vi "readAmbient.vi"() -> ()   [LabVIEW 2011]
uses:
  <vilib>/Utility/file.llb/Read From Spreadsheet File (string).vi
panel:
  out "Table Control":string[][](table)
  in  "EXIT":bool
  in  "OK Button":bool
  in  "Boolean":bool caption="Choose date    Today"
  out "Diff Press":cluster{dbl[], dbl[]}(graph)
  out "Press":cluster{dbl[], dbl[]}(graph)
  out "Umidity":cluster{dbl[], dbl[]}[](graph)=[{[1.0, 2.0, 4.0], [2.0, 1.0, 0.0]}, {[0.5, 1.5, 3.5], [3.0, 4.0, 2.0]}]
  out "Temperature":cluster{dbl[], dbl[]}[](graph)=[{[1.0, 2.0, 4.0], [2.0, 1.0, 0.0]}, {[0.5, 1.5, 3.5], [3.0, 4.0, 2.0]}]
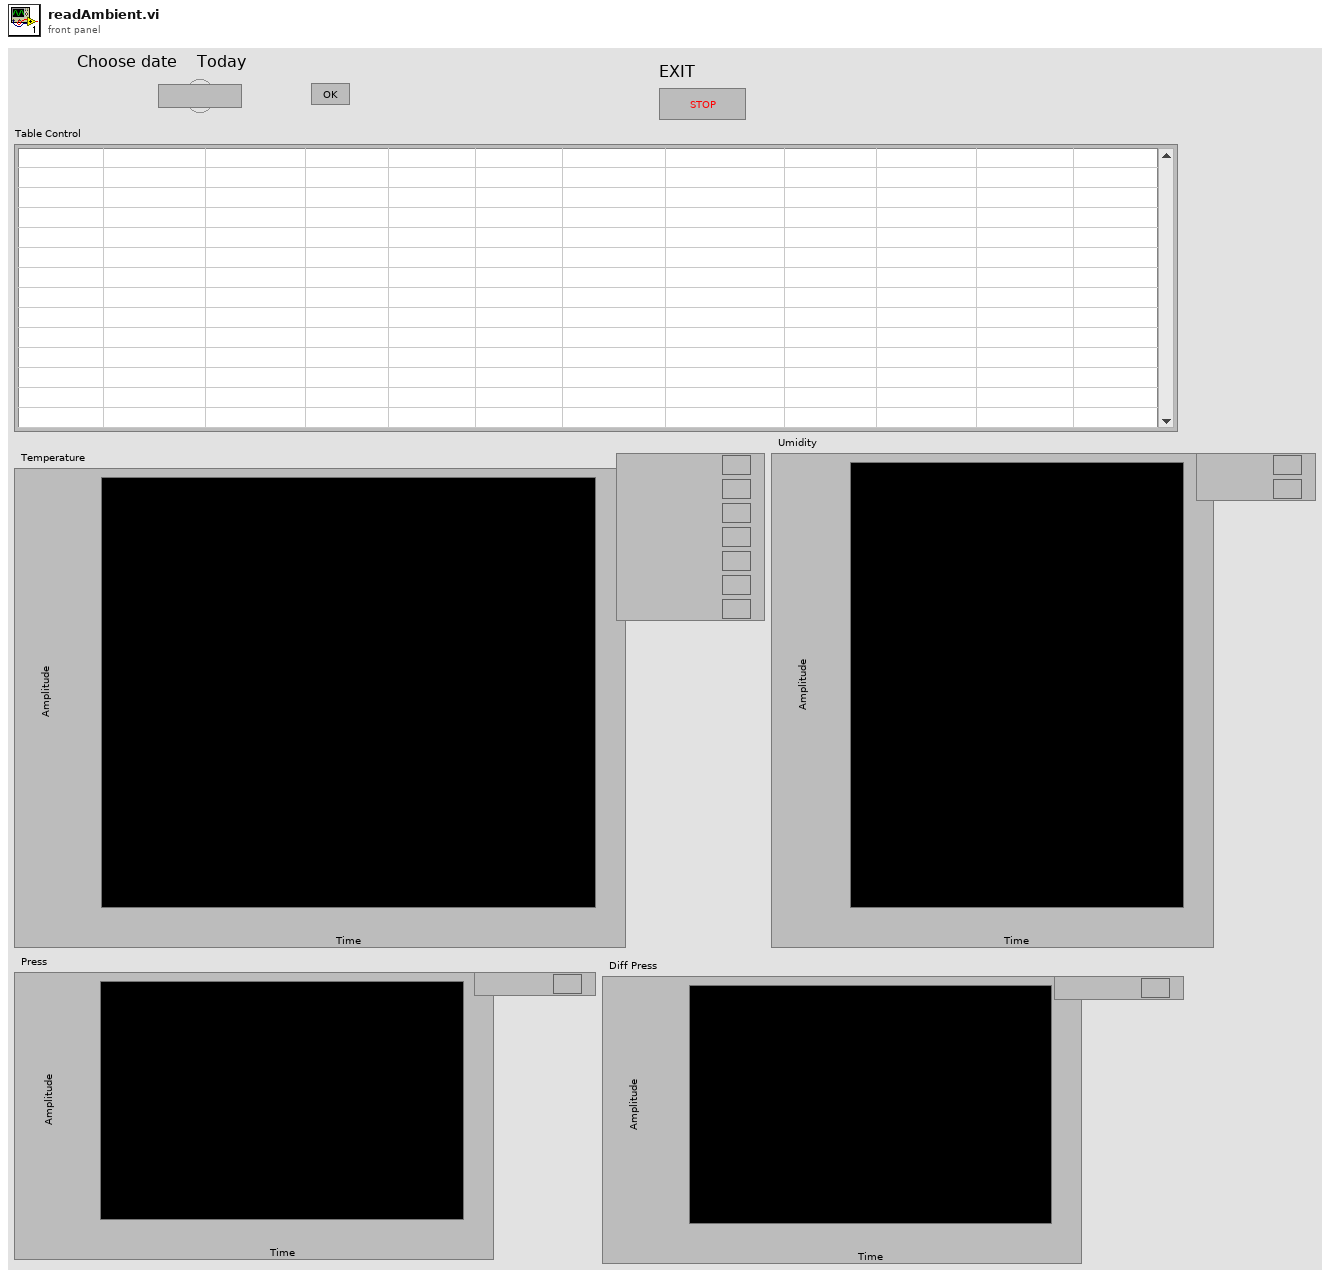
[diagram p1: front panel]
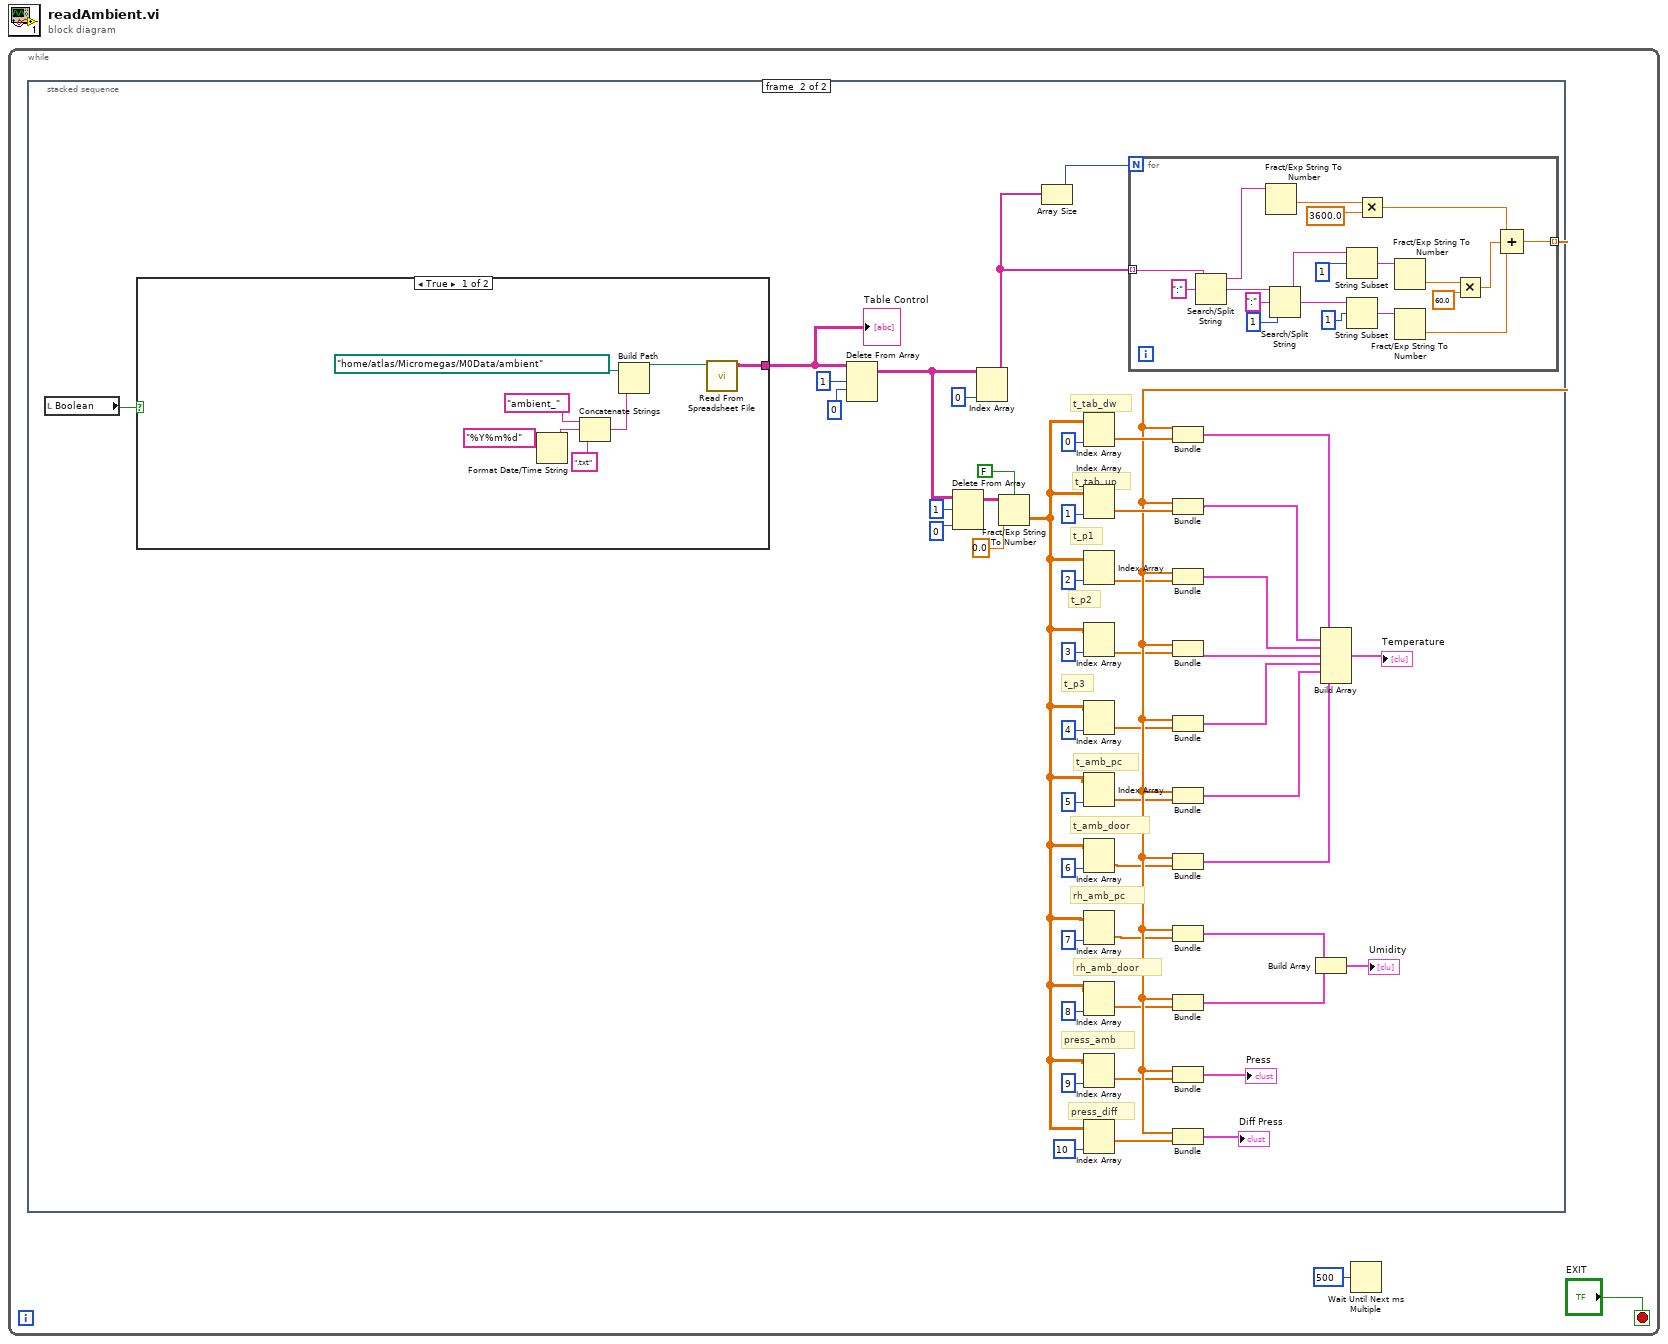
[diagram p0: block diagram]
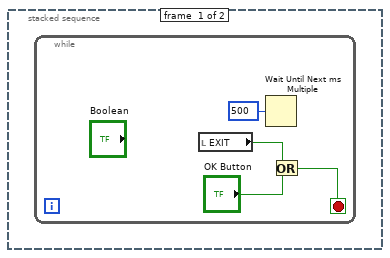
[diagram p2: hidden frame]
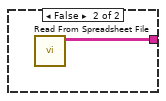
[diagram p3: hidden frame]
diagram:
  n1 = while {
    stop <- "EXIT" stop-if-true
    n2 = stacked-sequence {
      frame #0 {
        n3 = while {
          stop <- w3 stop-if-true
          n4 = local read "EXIT"() -> (w5:bool)
          n5 = Wait Until Next ms Multiple(millisecond multiple=u32 500) -> ()  [unwired: 1 out]
          n6 = Or(x=w5, y="OK Button") -> (x .or. y?=w3:bool)
        }
      }
      frame #1 {
        # "press_diff"
        # "press_amb"
        # "rh_amb_door"
        # "rh_amb_pc"
        # "t_amb_door"
        # "t_amb_pc"
        # "t_p3"
        # "t_p2"
        # "t_p1"
        # "t_tab_up"
        # "t_tab_dw"
        n7 = local read "Boolean"() -> (w8:bool)
        n8 = case shown="True" w8 {
          tunnel: [w59 w65] -> w7
          frame True {
            n9 = Format Date/Time String(time format string (%c)="%Y%m%d") -> (date/time string=w62:string)  [unwired: 2 in]
            n10 = Concatenate Strings("ambient_" ("string"), w62, ".txt" ("string")) -> (w60:string)
            n11 = Build Path(base path=path "/home/atlas/Micromegas/M0Data/ambient", name or relative path=w60) -> (appended path=w57:path)
            n12 = call-poly <vilib>:"Read From Spreadsheet File.vi"("file path (dialog if empty)"=w57) -> ("all rows"=w59:string[][])  [unwired: 6 in, 4 out]
          }
          frame False {
            n13 = call-poly <vilib>:"Read From Spreadsheet File.vi"() -> ("all rows"=w65:string[][])  [unwired: 7 in, 4 out]
          }
        }
        "Table Control" <- w7
        n14 = Delete From Array(array=w7, length=1, index (row)=0) -> (array with subset deleted=w50:string[][])  [unwired: 1 in, 1 out]
        n15 = Delete From Array(array=w50, length=1, index (col)=0 ("disabled index (col)")) -> (array with subset deleted=w53:string[][])  [unwired: 1 in, 1 out]
        n16 = Index Array(array=w50, index (col)=0 ("disabled index (col)")) -> (element=w51:string[])  [unwired: 1 in]
        n17 = Fract/Exp String To Number(use system decimal point (T)=FALSE, string=w53, default (0 dbl)=0.0 ("default (0 DBL)")) -> (number=w32:dbl[][])  [unwired: 1 in, 1 out]
        n18 = Array Size(array=w51) -> (size(s)=w52:i32)
        n19 = Index Array(array=w32, index (col)=0 ("disabled index (col)")) -> (element=w45:dbl[])  [unwired: 1 in]
        n20 = Index Array(array=w32, index (col)=1 ("disabled index (col)")) -> (element=w44:dbl[])  [unwired: 1 in]
        n21 = Index Array(array=w32, index (col)=2 ("disabled index (col)")) -> (element=w30:dbl[])  [unwired: 1 in]
        n22 = Index Array(array=w32, index (col)=3 ("disabled index (col)")) -> (element=w29:dbl[])  [unwired: 1 in]
        n23 = Index Array(array=w32, index (col)=4 ("disabled index (col)")) -> (element=w28:dbl[])  [unwired: 1 in]
        n24 = Index Array(array=w32, index (col)=5 ("disabled index (col)")) -> (element=w27:dbl[])  [unwired: 1 in]
        n25 = Index Array(array=w32, index (col)=6 ("disabled index (col)")) -> (element=w26:dbl[])  [unwired: 1 in]
        n26 = Index Array(array=w32, index (col)=7 ("disabled index (col)")) -> (element=w25:dbl[])  [unwired: 1 in]
        n27 = Index Array(array=w32, index (col)=8 ("disabled index (col)")) -> (element=w24:dbl[])  [unwired: 1 in]
        n28 = Index Array(array=w32, index (col)=9 ("disabled index (col)")) -> (element=w23:dbl[])  [unwired: 1 in]
        n29 = Index Array(array=w32, index (col)=10 ("disabled index (col)")) -> (element=w22:dbl[])  [unwired: 1 in]
        n30 = for {
          N: w52 -> [_]
          tunnel: w51 -> [w85] mode=indexing
          tunnel: [w77] -> w31 mode=indexing
          n31 = Search/Split String(string=w85, search string/char (-)=":") -> (substring before match=w81:string, match + rest of string=w82:string)  [unwired: 1 in, 1 out]
          n32 = Fract/Exp String To Number(string=w81) -> (number=w69:dbl)  [unwired: 3 in, 1 out]
          n33 = Search/Split String(string=w82, search string/char (-)=":", offset (0)=1) -> (substring before match=w75:string, match + rest of string=w71:string)  [unwired: 1 out]
          n34 = String Subset(string=w75, offset (0)=1) -> (substring=w73:string)  [unwired: 1 in]
          n35 = String Subset(string=w71, offset (0)=1) -> (substring=w70:string)  [unwired: 1 in]
          n36 = Multiply(x=w69, y=3600.0) -> (x*y=w68:dbl)
          n37 = Fract/Exp String To Number(string=w73) -> (number=w78:dbl)  [unwired: 3 in, 1 out]
          n38 = Fract/Exp String To Number(string=w70) -> (number=w66:dbl)  [unwired: 3 in, 1 out]
          n39 = Multiply(x=w78, y=60.0) -> (x*y=w67:dbl)
          n40 = Compound Arithmetic op=ADD(w68, w67, w66) -> (w77:dbl)
        }
        n41 = Bundle(w31, w45) -> (w21:cluster{dbl[], dbl[]})  [unwired: 1 in]
        n42 = Bundle(w31, w44) -> (w20:cluster{dbl[], dbl[]})  [unwired: 1 in]
        n43 = Bundle(w31, w30) -> (w19:cluster{dbl[], dbl[]})  [unwired: 1 in]
        n44 = Bundle(w31, w29) -> (w18:cluster{dbl[], dbl[]})  [unwired: 1 in]
        n45 = Bundle(w31, w28) -> (w17:cluster{dbl[], dbl[]})  [unwired: 1 in]
        n46 = Bundle(w31, w27) -> (w16:cluster{dbl[], dbl[]})  [unwired: 1 in]
        n47 = Bundle(w31, w26) -> (w15:cluster{dbl[], dbl[]})  [unwired: 1 in]
        n48 = Bundle(w31, w25) -> (w13:cluster{dbl[], dbl[]})  [unwired: 1 in]
        n49 = Bundle(w31, w24) -> (w12:cluster{dbl[], dbl[]})  [unwired: 1 in]
        n50 = Bundle(w31, w23) -> (→"Press":cluster{dbl[], dbl[]})  [unwired: 1 in]
        n51 = Bundle(w31, w22) -> (→"Diff Press":cluster{dbl[], dbl[]})  [unwired: 1 in]
        n52 = Build Array(w13, w12) -> (→"Umidity":cluster{dbl[], dbl[]}[])
        n53 = Build Array(w21, w20, w19, w18, w17, w16, w15) -> (→"Temperature":cluster{dbl[], dbl[]}[])
      }
    }
    n54 = Wait Until Next ms Multiple(millisecond multiple=u32 500) -> ()  [unwired: 1 out]
  }
